vi "GetVirtualChannelProperties.vi"(9 "channels":T2[](array[typedef]), 10 "channel":T2, 11 "tdms properties in":T1[](array[typedef])) -> (3 "tdms properties out":T1[](array[typedef]))   [LabVIEW 2017, in "Tdms.lvlib"]
uses:
  <vilib>/addons/InsightCM/Utilities/Tdms/Tdms.lvlib
  <vilib>/addons/InsightCM/MessageBus/Base/controls/R2_Channel.ctl
  <vilib>/addons/InsightCM/MessageBus/Base/controls/KeyValuePair.ctl
  <vilib>/addons/InsightCM/MessageBus/Base/controls/Metric.ctl
  <vilib>/addons/InsightCM/Utilities/Tdms/controls/Property.ctl
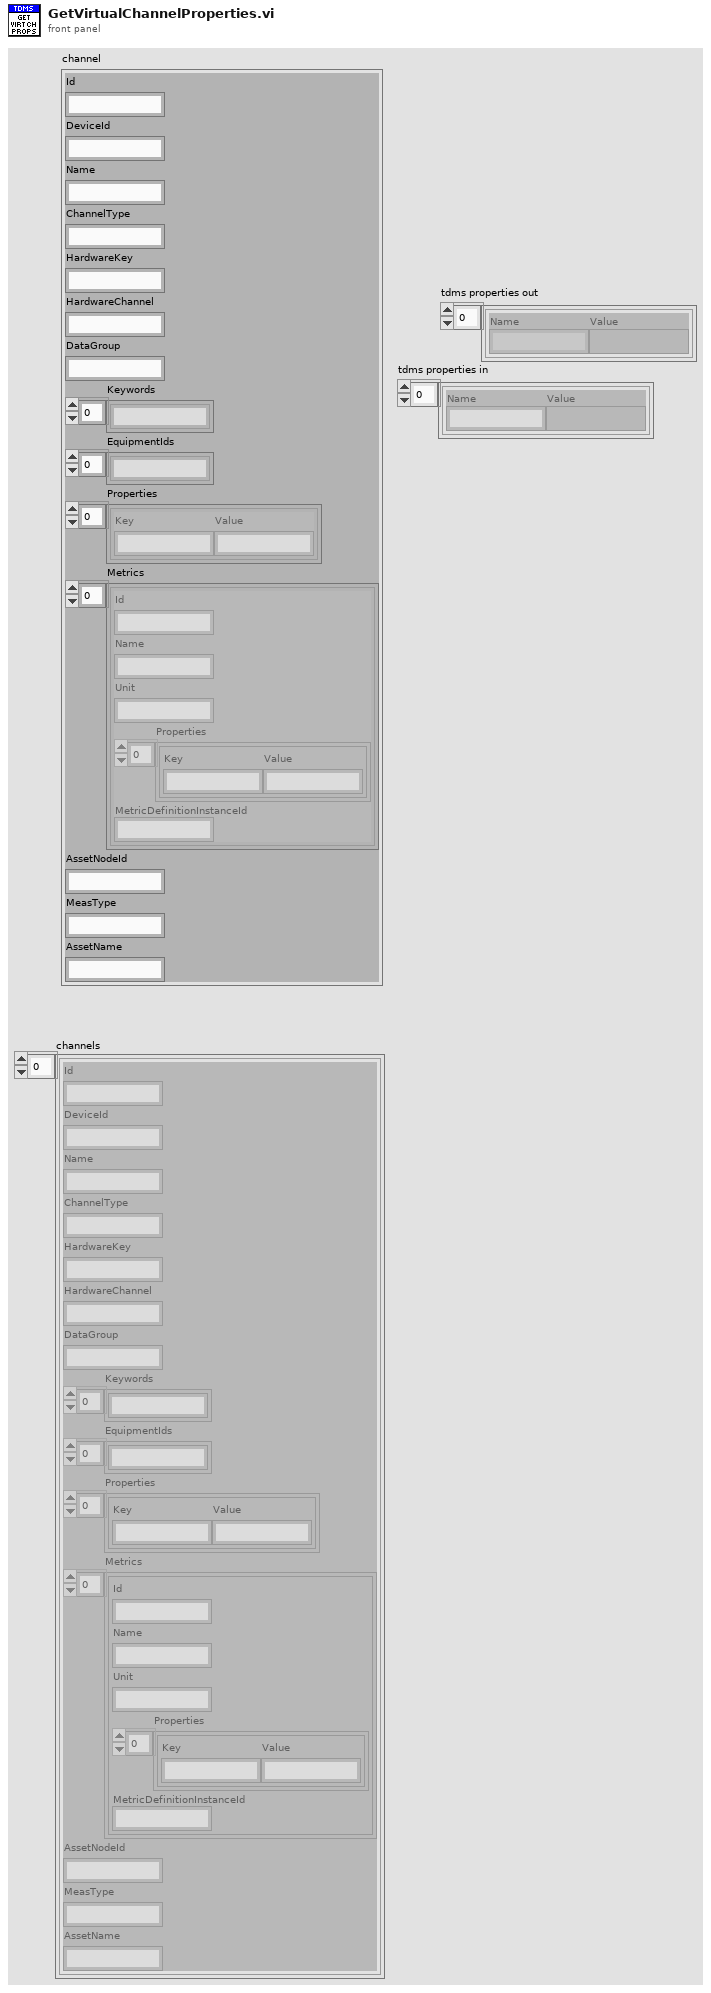
[diagram p1: front panel]
types:
  T1 = typedef "Tdms.lvlib/Property.ctl" = cluster{"Name":string, "Value":variant}
  T2 = typedef "R2_Channel.ctl" = cluster{"Id":string, "DeviceId":string, "Name":string, "ChannelType":string, "HardwareKey":string, "HardwareChannel":string, "DataGroup":string, "Keywords":string[], "EquipmentIds":string[], "Properties":T3[], "Metrics":T4[], "AssetNodeId":string, "MeasType":string, "AssetName":string}
  T3 = typedef "KeyValuePair.ctl" = cluster{"Key":string, "Value":string}
  T4 = typedef "Metric.ctl" = cluster{"Id":string, "Name":string, "Unit":string, "Properties":T3[], "MetricDefinitionInstanceId":string}
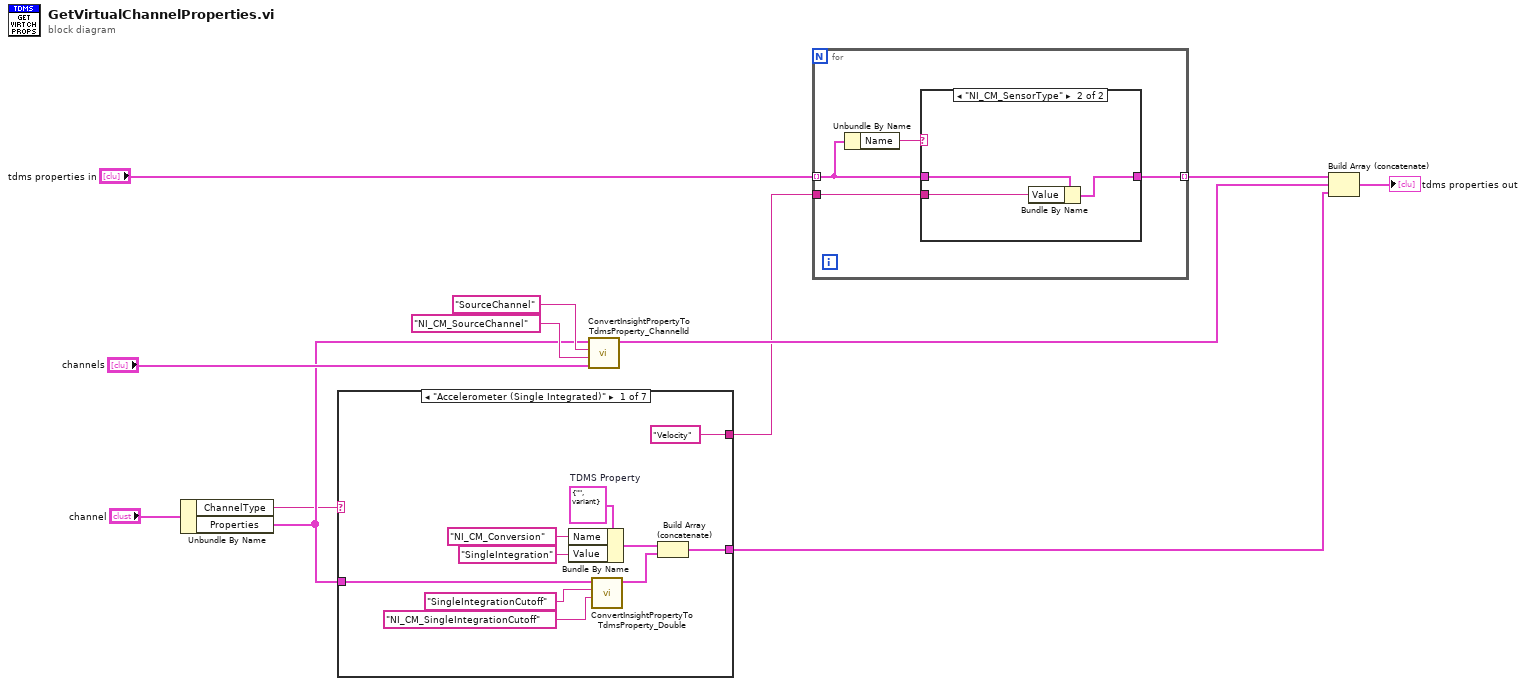
[diagram p0: block diagram]
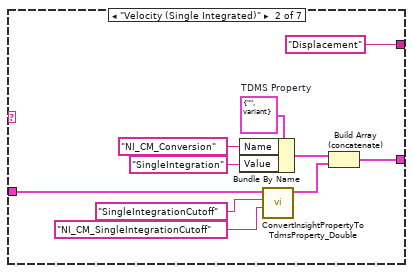
[diagram p3: hidden frame]
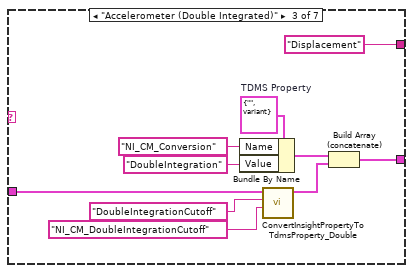
[diagram p4: hidden frame]
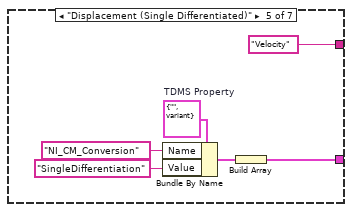
[diagram p6: hidden frame]
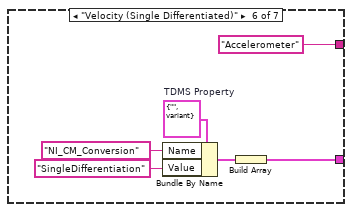
[diagram p7: hidden frame]
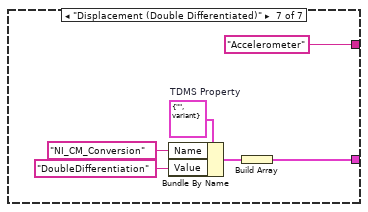
[diagram p8: hidden frame]
diagram:
  n1 = Unbundle By Name("channel") -> ("ChannelType"=w7:string, "Properties"=w8:T3[])
  n2 = case shown="\"Accelerometer (Single Integrated)\"" w7 {
    tunnel: [w15 w25 w40 _ w44 w50 w56] -> w3
    tunnel: w8 -> [w14 w24 w37 _ _ _ _]
    tunnel: ["Velocity" ("Name") "Displacement" ("Name") "Displacement" ("Name") _ "Velocity" ("Name") "Accelerometer" ("Name") "Accelerometer" ("Name")] -> w2
    frame "Accelerometer (Single Integrated)" {
      w19 = T1 {"Name"="", "Value"=variant}  # TDMS Property
      n3 = Bundle By Name(cluster=w19, "Name"="NI_CM_Conversion", "Value"="SingleIntegration" ("Name")) -> (w21:T1)
      n4 = call <vilib>:"ConvertInsightPropertyToTdmsProperty_Double.vi"("Tdms Property Name"="NI_CM_SingleIntegrationCutoff" ("Name"), "Insight Property Name"="SingleIntegrationCutoff" ("Name"), "Insight Properties"=w14) -> ("Tdms Properties"=w18:T1[])  [unwired: 8 in]
      n5 = Build Array (concatenate)(w21, w18) -> (w15:T1[])
    }
    frame "Velocity (Single Integrated)" {
      w29 = T1 {"Name"="", "Value"=variant}  # TDMS Property
      n6 = Bundle By Name(cluster=w29, "Name"="NI_CM_Conversion", "Value"="SingleIntegration" ("Name")) -> (w31:T1)
      n7 = call <vilib>:"ConvertInsightPropertyToTdmsProperty_Double.vi"("Tdms Property Name"="NI_CM_SingleIntegrationCutoff" ("Name"), "Insight Property Name"="SingleIntegrationCutoff" ("Name"), "Insight Properties"=w24) -> ("Tdms Properties"=w28:T1[])  [unwired: 8 in]
      n8 = Build Array (concatenate)(w31, w28) -> (w25:T1[])
    }
    frame "Accelerometer (Double Integrated)" {
      w38 = T1 {"Name"="", "Value"=variant}  # TDMS Property
      n9 = Bundle By Name(cluster=w38, "Name"="NI_CM_Conversion", "Value"="DoubleIntegration" ("Name")) -> (w41:T1)
      n10 = call <vilib>:"ConvertInsightPropertyToTdmsProperty_Double.vi"("Tdms Property Name"="NI_CM_DoubleIntegrationCutoff" ("Name"), "Insight Property Name"="DoubleIntegrationCutoff" ("Name"), "Insight Properties"=w37) -> ("Tdms Properties"=w36:T1[])  [unwired: 8 in]
      n11 = Build Array (concatenate)(w41, w36) -> (w40:T1[])
    }
    frame Default {
    }
    frame "Displacement (Single Differentiated)" {
      w46 = T1 {"Name"="", "Value"=variant}  # TDMS Property
      n12 = Bundle By Name(cluster=w46, "Name"="NI_CM_Conversion", "Value"="SingleDifferentiation" ("Name")) -> (w45:T1)
      n13 = Build Array(w45) -> (w44:T1[])
    }
    frame "Velocity (Single Differentiated)" {
      w52 = T1 {"Name"="", "Value"=variant}  # TDMS Property
      n14 = Bundle By Name(cluster=w52, "Name"="NI_CM_Conversion", "Value"="SingleDifferentiation" ("Name")) -> (w51:T1)
      n15 = Build Array(w51) -> (w50:T1[])
    }
    frame "Displacement (Double Differentiated)" {
      w58 = T1 {"Name"="", "Value"=variant}  # TDMS Property
      n16 = Bundle By Name(cluster=w58, "Name"="NI_CM_Conversion", "Value"="DoubleDifferentiation" ("Name")) -> (w57:T1)
      n17 = Build Array(w57) -> (w56:T1[])
    }
  }
  n18 = call <vilib>:"ConvertInsightPropertyToTdmsProperty_ChannelId.vi"("Insight Channels"="channels", "Tdms Property Name"="NI_CM_SourceChannel" ("Name"), "Insight Property Name"="SourceChannel" ("name"), "Insight Properties"=w8) -> ("Tdms Properties"=w4:T1[])  [unwired: 7 in]
  n19 = for {
    tunnel: "tdms properties in" -> [w62] mode=indexing
    tunnel: [w63] -> w5 mode=indexing
    tunnel: w2 -> [w61]
    n20 = Unbundle By Name(w62) -> ("Name"=w64:string)
    n21 = case shown="\"NI_CM_SensorType\"" w64 {
      tunnel: [w65 w67] -> w63
      tunnel: w62 -> [w65 w68]
      tunnel: w61 -> [_ w66]
      frame Default {
      }
      frame "NI_CM_SensorType" {
        n22 = Bundle By Name(cluster=w68, "Value"=w66) -> (w67:T1)
      }
    }
  }
  n23 = Build Array (concatenate)(w5, w4, w3) -> (→"tdms properties out":T1[])
